vi "Airpuff-Init.vi"(7 "Device reference":refnum<vi>, 8 "error in (no error)":errorcluster, 10 "OutputRequest event ref":T1, 11 "InputData reference":refnum<vi>) -> (0 "error out":errorcluster, 2 "OutputRequest (dup)":T1, 3 "InputData (dup)":refnum<vi>)   [LabVIEW 2015]
doc: "Initializes a valve object. Wire its reference to the \"Device reference\" input.\n\nInputData reference: create reference from Main VI\nOutputRequest event ref: get this from Rack-Init\n\nThe outputs are just duplicates to make it easier to call a bunch of Device-Init functions."
uses:
  Rack/Typedefs/OutputRequest refnum.ctl
  Rack/Typedefs/OutputRequest.ctl
  Rack/Typedefs/InputData cluster.ctl
  Rack/Methods/Port drivers/DigitalInput-DataCluster.ctl
  Typedefs/Speaker.ctl
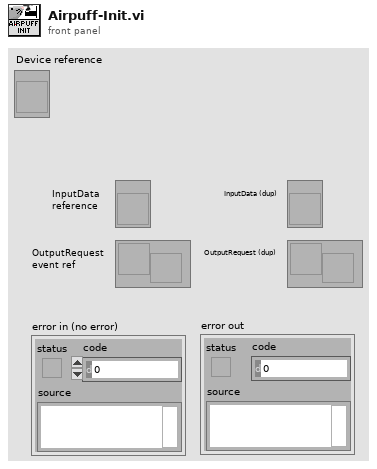
[diagram p1: front panel]
types:
  T1 = typedef "OutputRequest refnum.ctl" = refnum<user-event>
  T2 = typedef "Speaker.ctl" = cluster{"Settings":cluster{"Portname":string, "Index":i32, "Timestamp portname":string}, "OutputRequest event ref":T1, "InputData reference":refnum<vi>}
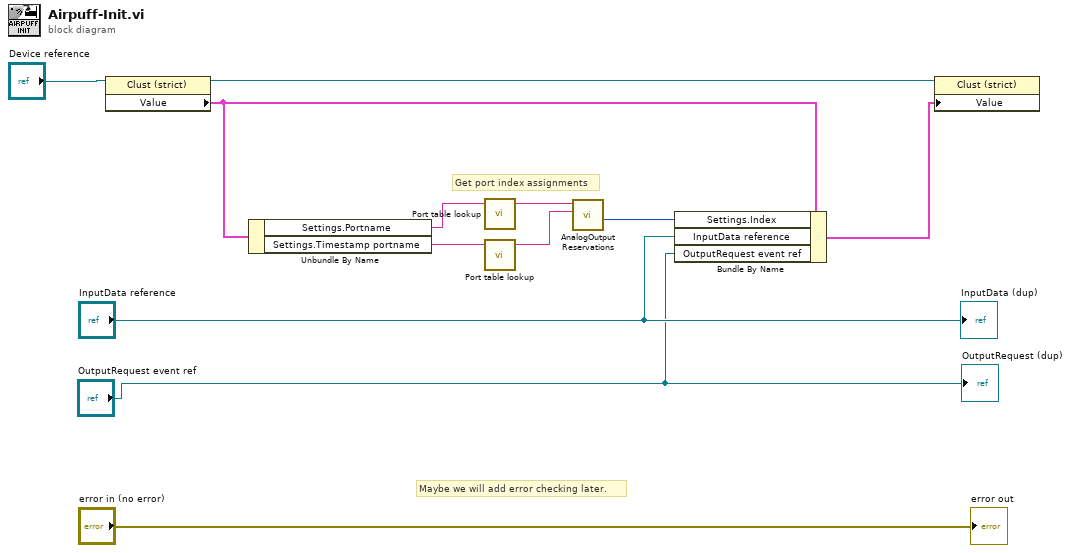
[diagram p0: block diagram]
diagram:
  # "Get port index assignments"
  # "Maybe we will add error checking later."
  n1 = property class="Clust (strict)"(reference="Device reference") -> (reference out=w12:refnum<vi>, "Value"=w5:T2)  [unwired: 1 in, 1 out]
  n2 = Unbundle By Name(w5) -> ("Settings.Portname"=w9:string, "Settings.Timestamp portname"=w8:string)
  n3 = call "Port table lookup.vi"("Port name"=w9) -> ("Line"=w11:tag)  [unwired: 3 in, 1 out]
  n4 = call "Port table lookup.vi"("Port name"=w8) -> ("Line"=w7:tag)  [unwired: 3 in, 1 out]
  n5 = call "AnalogOutput Reservations.vi"("Timestamp line"=w7, "Line"=w11) -> ("Index assigned"=w10:i32)  [unwired: 2 in, 3 out]
  n6 = Bundle By Name(cluster=w5, "Settings.Index"=w10, "InputData reference"="InputData reference", "OutputRequest event ref"="OutputRequest event ref") -> (w4:T2)
  n7 = property class="Clust (strict)"(reference=w12, "Value"=w4) -> ()  [unwired: 1 in, 2 out]
  "error out" <- "error in (no error)"
  "OutputRequest (dup)" <- "OutputRequest event ref"
  "InputData (dup)" <- "InputData reference"
